vi "Serve_Current_Time.vi"(11 "LabVIEW Web Service Request":refnum<class "Web Request.lvclass">) -> ()   [LabVIEW 2013]
uses:
  <vilib>/wsapi/Web Request.lvclass
  <vilib>/xml/Close Reference(Node).vi
  <vilib>/xml/NI_XML.lvlib
  <resource>/objmgr/DOMUserDefRef.rc
panel:
  out "XML":string
  out "*(type *) &x":dbl format="%.2f"
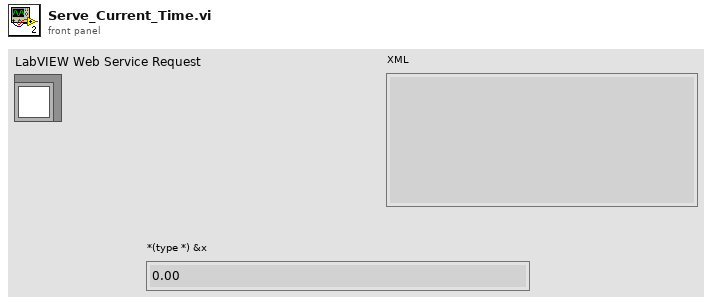
[diagram p1: front panel]
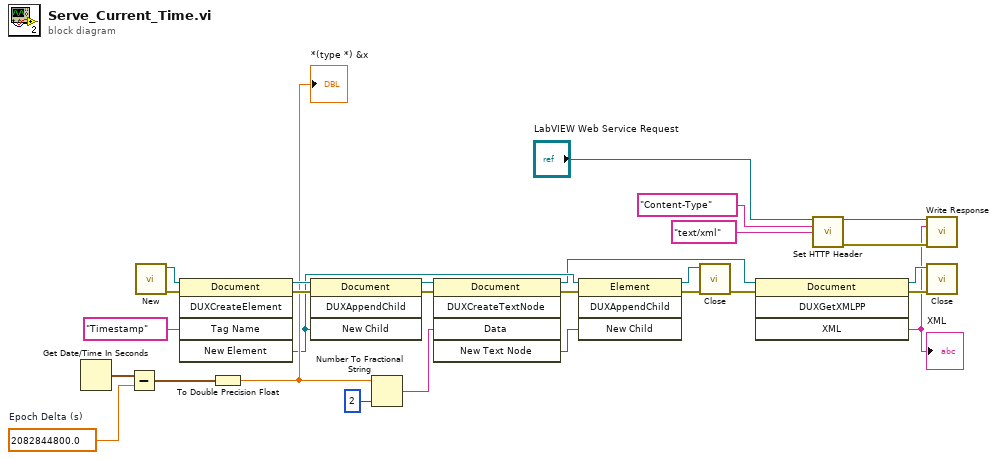
[diagram p0: block diagram]
diagram:
  w1 = 2082844800.0  # Epoch Delta (s)
  n1 = Get Date/Time In Seconds() -> (seconds since 1Jan1904=w28:timestamp)
  n2 = Subtract(x=w28, y=w1) -> (x-y=w27:timestamp)
  n3 = call <vilib>:"New.vi"() -> ("error out"=w25:errorcluster, "DOM document out"=w26:refnum<k20>)  [unwired: 8 in]
  n4 = invoke class="Document" method="DUXCreateElement"(reference=w26, error in=w25, "Tag Name"="Timestamp") -> (reference out=w23:refnum<k20>, error out=w22:errorcluster, "New Element"=w17:refnum<k20>)  [unwired: 2 in, 2 out]
  n5 = To Double Precision Float(number=w27) -> (double precision float=w20:dbl)
  "*(type *) &x" <- w20
  n6 = invoke class="Document" method="DUXAppendChild"(reference=w23, error in=w22, "New Child"=w17) -> (reference out=w21:refnum<k20>, error out=w12:errorcluster)  [unwired: 1 in, 2 out]
  n7 = Number To Fractional String(number=w20, precision (6)=i16 2) -> (F-format string=w18:string)  [unwired: 2 in]
  n8 = invoke class="Document" method="DUXCreateTextNode"(reference=w21, error in=w12, "Data"=w18) -> (reference out=w11:refnum<k20>, error out=w16:errorcluster, "New Text Node"=w15:refnum<k20>)  [unwired: 2 in, 2 out]
  n9 = invoke class="Element" method="DUXAppendChild"(reference=w17, error in=w16, "New Child"=w15) -> (reference out=w13:refnum<k20>, error out=w14:errorcluster)  [unwired: 1 in, 2 out]
  n10 = call-poly <vilib>:"Close.vi"("error in (no error)"=w14, "node"=w13) -> ("error out"=w9:errorcluster)  [unwired: 7 in]
  n11 = invoke class="Document" method="DUXGetXMLPP"(reference=w11, error in=w9) -> (reference out=w10:refnum<k20>, error out=w8:errorcluster, "XML"=w2:string)  [unwired: 2 in, 1 out]
  "XML" <- w2
  n12 = call <vilib>:"Set HTTP Header.vi"("LabVIEW Web Service Request"="LabVIEW Web Service Request", "header"="Content-Type", "header value"="text/xml") -> ("LabVIEW Web Service Request out"=w6:refnum<class "Web Request.lvclass">, "error out"=w5:errorcluster)  [unwired: 11 in]
  n13 = call <vilib>:"Write Response.vi"("LabVIEW Web Service Request"=w6, "response string"=w2, "error in (no error)"=w5) -> ()  [unwired: 11 in, 2 out]
  n14 = call-poly <vilib>:"Close.vi"("error in (no error)"=w8, "node"=w10) -> ()  [unwired: 7 in, 1 out]
